vi "escape.vi"(7 "type":T1, 11 "string":string) -> (3 "escaped":string)   [LabVIEW 2013, in "uniform resource locator.lvlib"]
uses:
  uniform resource locator.lvlib
  encoding type.ctl
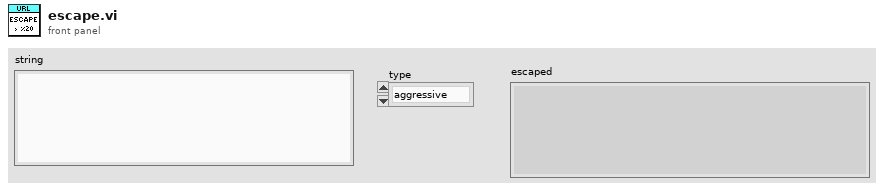
[diagram p1: front panel]
types:
  T1 = typedef "uniform resource locator.lvlib/encoding type.ctl" = enum16{"aggressive", "path segment", "full path", "query", "fragment"}
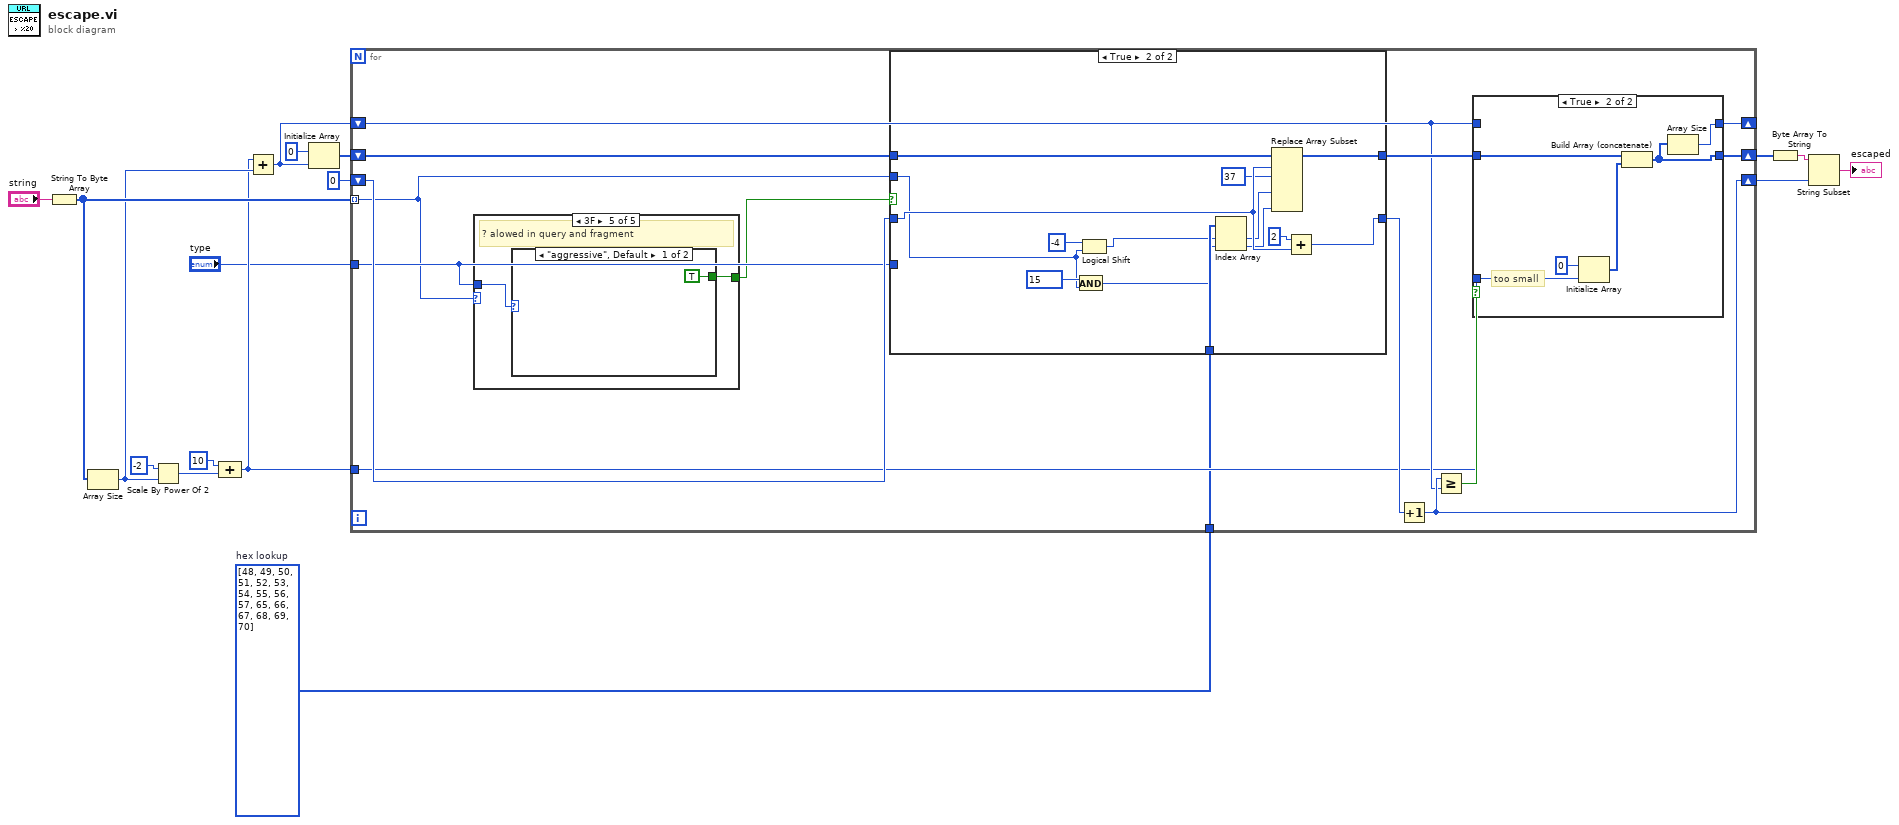
[diagram p0: block diagram]
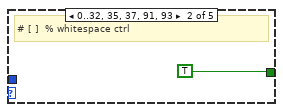
[diagram p3: hidden frame]
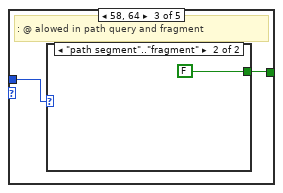
[diagram p4: hidden frame]
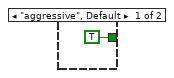
[diagram p5: hidden frame]
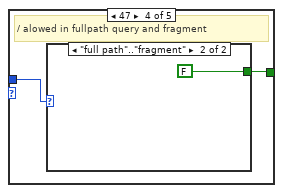
[diagram p6: hidden frame]
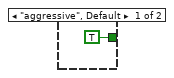
[diagram p7: hidden frame]
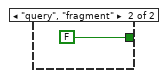
[diagram p8: hidden frame]
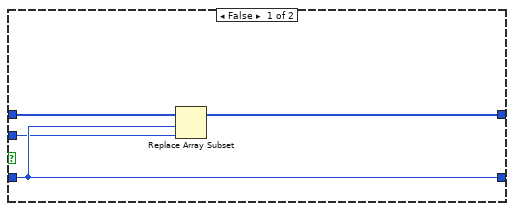
[diagram p10: hidden frame]
diagram:
  w2 = u8[] [48, 49, 50, 51, 52, 53, 54, 55, 56, 57, 65, 66, 67, 68, 69, 70]  # hex lookup
  n1 = String To Byte Array(string="string") -> (unsigned byte array=w7:u8[])
  n2 = Array Size(array=w7) -> (size(s)=w4:i32)
  n3 = Scale By Power Of 2(n=i16 -2, x=w4) -> (x*2^n=w11:i32)
  n4 = Compound Arithmetic op=ADD(10 ("value"), w11) -> (w3:i32)
  n5 = Add(x=w3, y=w4) -> (x+y=w5:i32)
  n6 = Initialize Array(u8 0 ("value"), w5) -> (w8:u8[])
  n7 = for {
    shift-right: [w28] -> w13
    shift-left: 0 -> [w31]
    shift-right: [w26] -> w6
    shift-left: w8 -> [w30]
    tunnel: w7 -> [w18] mode=indexing
    shift-right: [w23] -> _
    shift-left: w5 -> [w24]
    tunnel: w3 -> [w22]
    tunnel: w2 -> [w21]
    tunnel: "type" -> [w20]
    n8 = case shown="3F" w18 {
      tunnel: [_ TRUE w34 w38 w42] -> w19
      tunnel: w20 -> [_ _ w33 w37 w41]
      frame Default {
      }
      frame 0..32, 35, 37, 91, 93 {
        # "# [ ]  % whitespace ctrl"
      }
      frame 58, 64 {
        # ": @ alowed in path query and fragment"
        n9 = case shown="\"path segment\"..\"fragment\"" w33 {
          tunnel: [TRUE FALSE] -> w34
          frame "aggressive", Default {
          }
          frame "path segment".."fragment" {
          }
        }
      }
      frame 47 {
        # "/ alowed in fullpath query and fragment"
        n10 = case shown="\"full path\"..\"fragment\"" w37 {
          tunnel: [TRUE FALSE] -> w38
          frame "aggressive", Default {
          }
          frame "full path".."fragment" {
          }
        }
      }
      frame 63 {
        # "? alowed in query and fragment"
        n11 = case shown="\"aggressive\", Default" w41 {
          tunnel: [TRUE FALSE] -> w42
          frame "aggressive", Default {
          }
          frame "query", "fragment" {
          }
        }
      }
    }
    n12 = case shown="True" w19 {
      tunnel: [w56 w70] -> w25
      tunnel: w31 -> [w54 w68]
      tunnel: w30 -> [w55 w69]
      tunnel: [w54 w67] -> w29
      tunnel: w21 -> [_ w60]
      tunnel: w20 -> [_ _]
      tunnel: w18 -> [w53 w57]
      frame False {
        n13 = Replace Array Subset(array=w55, new element=w53, index=w54) -> (w56:u8[])
      }
      frame True {
        # "# [ ]  % whitespace ctrl"
        n14 = And(x=u8 15, y=w57) -> (x .and. y?=w58:u8)
        n15 = Logical Shift(y=i16 -4, x=w57) -> (x << y=w59:u8)
        n16 = Index Array(array=w60, index #1=w59, index #2=w58) -> (element #1=w65:u8, element #2=w64:u8)
        n17 = Replace Array Subset(array=w69, new element #1=u8 37 ("new element/subarray"), index #1=w68, new element #2=w65, new element #3=w64) -> (w70:u8[])  [unwired: 2 in]
        n18 = Add(x=2, y=w68) -> (x+y=w67:i32)
      }
    }
    n19 = Increment(x=w29) -> (x+1=w28:i32)
    n20 = Greater Or Equal?(x=w28, y=w24) -> (x >= y?=w27:bool)
    n21 = case shown="True" w27 {
      tunnel: [w46 w47] -> w26
      tunnel: w25 -> [w46 w50]
      tunnel: w24 -> [w45 _]
      tunnel: [w45 w48] -> w23
      tunnel: w22 -> [_ w51]
      frame False {
        # "size ok"
      }
      frame True {
        # "too small"
        n22 = Initialize Array(u8 0 ("value"), w51) -> (w49:u8[])
        n23 = Build Array (concatenate)(w50, w49) -> (w47:u8[])
        n24 = Array Size(array=w47) -> (size(s)=w48:i32)
      }
    }
  }
  n25 = Byte Array To String(unsigned byte array=w6) -> (string=w15:string)
  n26 = String Subset(string=w15, length (rest)=w13) -> (substring=→"escaped":string)  [unwired: 1 in]
